vi "Acquire_PID_Tests_steps_gs.vi"() -> ()   [LabVIEW 2016]
uses:
  Globals/PressuresGlobal.vi
panel:
  in  "PID Time":dbl=20.0
  out "Current Set point":dbl
  out "Exp Time":dbl
  in  "Time_Stable(s)":dbl=20.0
  in  "Set Points":dbl[](array[numeric])=[0.1, 0.2, 0.3, 0.4, 0.5, 0.6, 0.7, 0.8, 0.9]
  in  "Wait For Microscope?":bool=TRUE
  in  "stop2":bool
  in  "Flow Path":path=path "E:/maggot images/Jacob/20171121/stepTest20units_run101.mat"
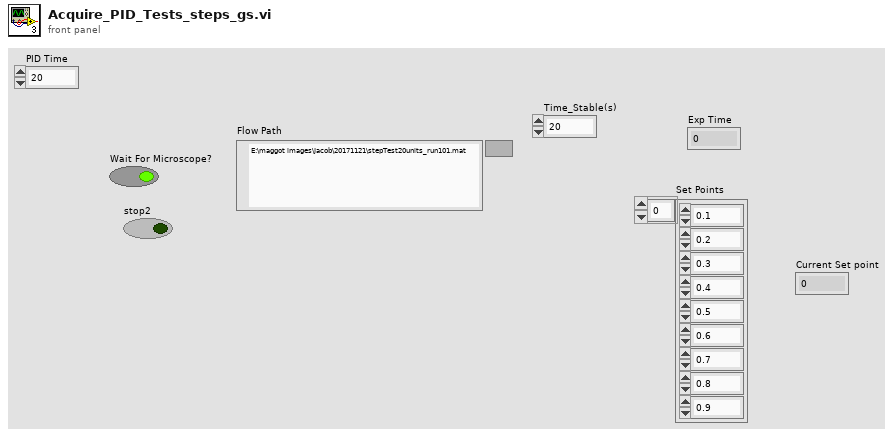
[diagram p1: front panel]
types:
  T1 = cluster{"relative seconds":dbl, "Pressures":dbl[], "F1 PID gains":dbl[], "FTot PID gains":dbl[], "PID On?":i16, "flow setpoints":dbl[]}
  T2 = cluster{"Time":dbl, "All Flow-Rates":dbl[], "Flow 2 Filter Time":dbl, "Flow 1 Filter Time":dbl}
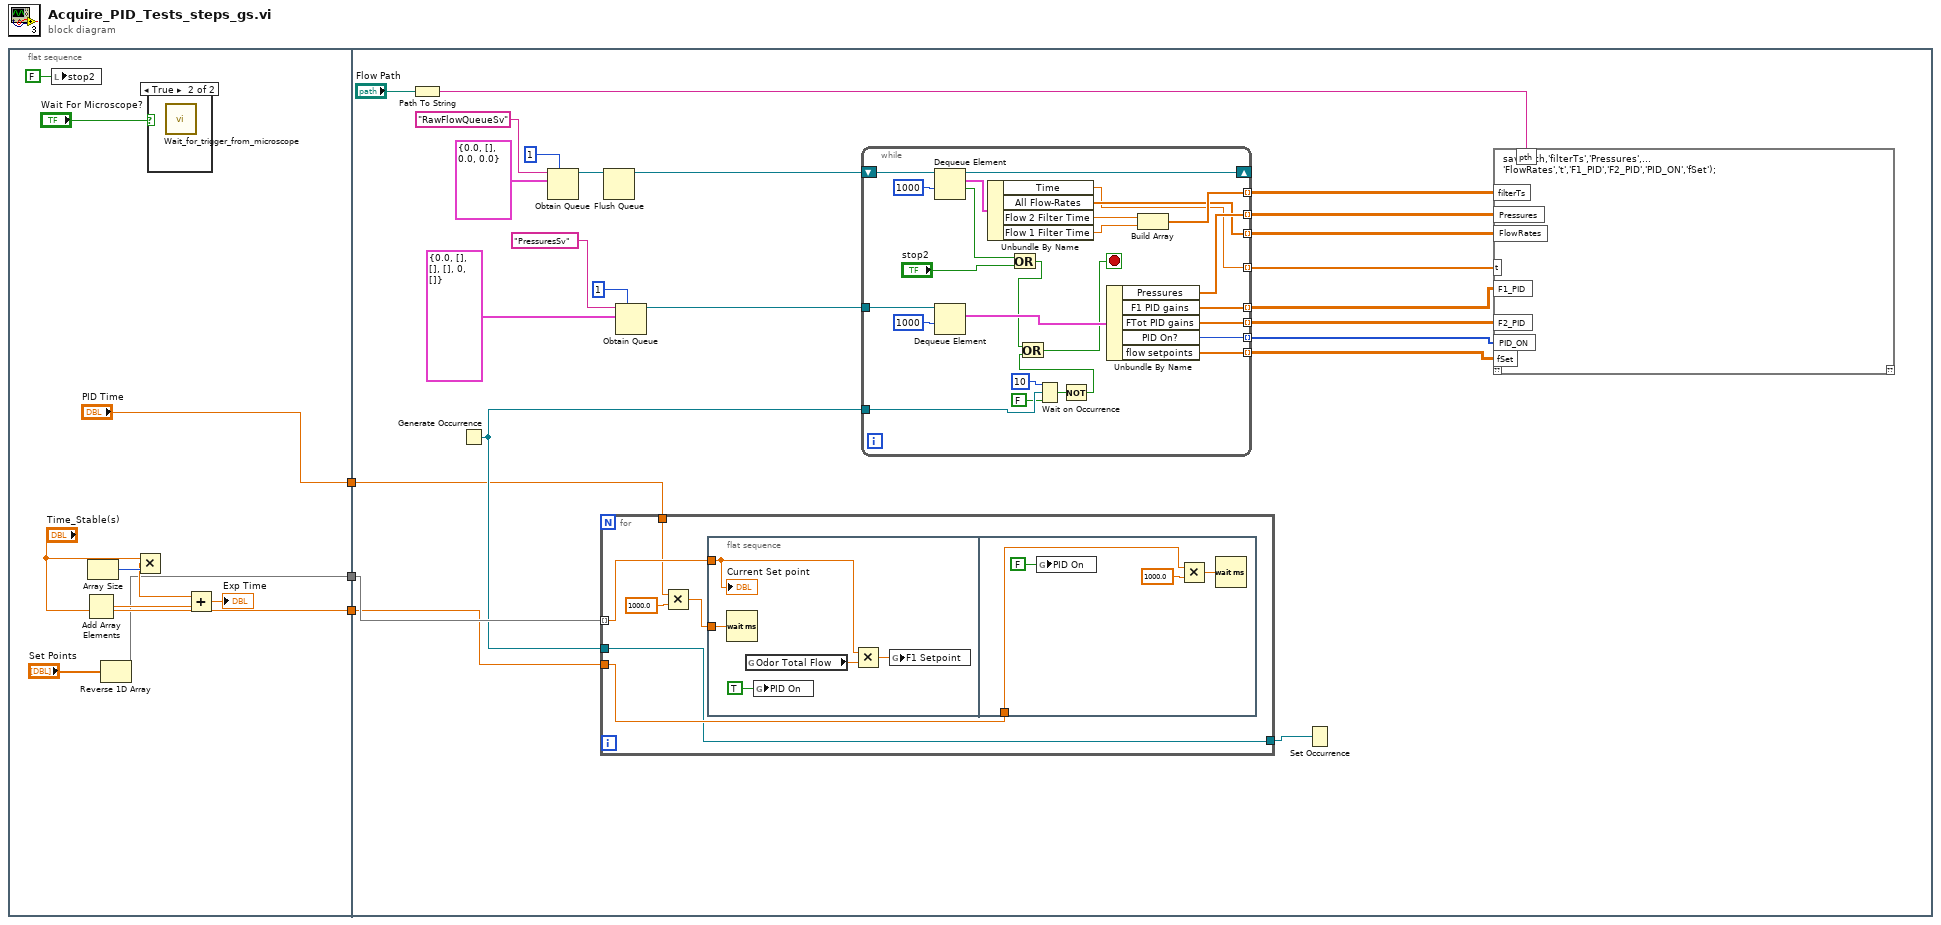
[diagram p0: block diagram]
diagram:
  n1 = flat-sequence {
    tunnel: [w5] -> w3
    tunnel: ["Time_Stable(s)"] -> w2
    tunnel: ["PID Time"] -> w1
    tunnel: w3 -> [w18]
    tunnel: w2 -> [w17]
    tunnel: w1 -> [w14]
    frame #0 {
      n2 = local write "stop2"(FALSE ("stop2")) -> ()
      n3 = Add Array Elements() -> (sum=w7:dbl)  [unwired: 1 in]
      n4 = Array Size() -> (size(s)=w9:i32)  [unwired: 1 in]
      n5 = Reverse 1D Array(array="Set Points") -> (reversed array=w5:dbl[])
      n6 = Multiply(x="Time_Stable(s)", y=w9) -> (x*y=w8:dbl)
      n7 = case shown="True" "Wait For Microscope?" {
        frame False {
        }
        frame True {
          n8 = call "Wait_for_trigger_from_microscope.vi"() -> ()  [unwired: 12 in]
        }
      }
      n9 = Add(x=w8, y=w7) -> (x+y=→"Exp Time":dbl)
    }
    frame #1 {
      n10 = Path To String(path="Flow Path") -> (string=w21:string)
      n11 = Generate Occurrence() -> (w16:refnum<k4>)
      n12 = Obtain Queue(max queue size (-1, unlimited)=1, name (unnamed)="RawFlowQueueSv", element data type=T2 {"Time"=0.0, "All Flow-Rates"=[], "Flow 2 Filter Time"=0.0, "Flow 1 Filter Time"=0.0} ("output cluster")) -> (queue out=w36:refnum<queue>)  [unwired: 2 in, 2 out]
      n13 = for {
        tunnel: w18 -> [w43] mode=indexing
        tunnel: w17 -> [w40]
        tunnel: w16 -> [w39]
        tunnel: [w39] -> w15
        tunnel: w14 -> [w38]
        n14 = Multiply(x=w38, y=1000.0) -> (x*y=w41:dbl)
        n15 = flat-sequence {
          tunnel: w43 -> [w47]
          tunnel: w41 -> [w45]
          tunnel: w40 -> [w50]
          frame #0 {
            n16 = Wait (ms)(milliseconds to wait=w45) -> ()  [unwired: 1 out]
            n17 = global read "PressuresGlobal.vi" "Odor Total Flow"() -> (w48:dbl)
            n18 = global write "PressuresGlobal.vi" "PID On"(TRUE ("PID On")) -> ()
            n19 = Multiply(x=w47, y=w48) -> (x*y=w46:dbl)
            n20 = global write "PressuresGlobal.vi" "F1 Setpoint"(w46) -> ()
            "Current Set point" <- w47
          }
          frame #1 {
            n21 = global write "PressuresGlobal.vi" "PID On"(FALSE ("PID On")) -> ()
            n22 = Multiply(x=w50, y=1000.0) -> (x*y=w51:dbl)
            n23 = Wait (ms)(milliseconds to wait=w51) -> ()  [unwired: 1 out]
          }
        }
      }
      n24 = Flush Queue(queue=w36) -> (queue out=w35:refnum<queue>)  [unwired: 1 in, 2 out]
      n25 = Obtain Queue(max queue size (-1, unlimited)=1, name (unnamed)="PressuresSv", element data type=T1 {"relative seconds"=0.0, "Pressures"=[], "F1 PID gains"=[], "FTot PID gains"=[], "PID On?"=0, "flow setpoints"=[]} ("output cluster")) -> (queue out=w31:refnum<queue>)  [unwired: 2 in, 2 out]
      n26 = while {
        shift-right: [w75] -> _
        shift-left: w35 -> [w78]
        tunnel: w31 -> [w72]
        tunnel: [w67] -> w22 mode=indexing
        tunnel: [w66] -> w23 mode=indexing
        tunnel: [w65] -> w24 mode=indexing
        tunnel: [w64] -> w26 mode=indexing
        tunnel: [w63] -> w28 mode=indexing
        tunnel: [w62] -> w27 mode=indexing
        tunnel: [w61] -> w25 mode=indexing
        tunnel: [w60] -> w19 mode=indexing
        tunnel: w16 -> [w59]
        stop <- w54 stop-if-true
        n27 = Dequeue Element(queue=w78, timeout in ms (-1)=1000) -> (queue out=w75:refnum<queue>, element=w71:T2, timed out?=w76:bool)  [unwired: 1 in, 1 out]
        n28 = Dequeue Element(queue=w72, timeout in ms (-1)=1000) -> (element=w68:T1)  [unwired: 1 in, 3 out]
        n29 = Unbundle By Name(w71) -> ("Time"=w61:dbl, "All Flow-Rates"=w62:dbl[], "Flow 2 Filter Time"=w70:dbl, "Flow 1 Filter Time"=w69:dbl)
        n30 = Or(x=w76, y="stop2") -> (x .or. y?=w55:bool)
        n31 = Wait on Occurrence(1:FALSE ("ignore previous (T)"), 2:w59, 3:10 ("ms timeout (-1)")) -> (0:w56:bool)
        n32 = Not(x=w56) -> (.not. x?=w53:bool)
        n33 = Or(x=w55, y=w53) -> (x .or. y?=w54:bool)
        n34 = Unbundle By Name(w68) -> ("Pressures"=w64:dbl[], "F1 PID gains"=w65:dbl[], "FTot PID gains"=w66:dbl[], "PID On?"=w67:i16, "flow setpoints"=w60:dbl[])
        n35 = Build Array(w70, w69) -> (w63:dbl[])
      }
      n36 = Set Occurrence(w15) -> ()
      n37 = script code="save(pth,'filterTs','Pressures',...\n'FlowRates','t','F1_PID','F2_PID','PID_ON','fSet');"("pth"=w21, "t"=w25, "F1_PID"=w24, "F2_PID"=w23, "PID_ON"=w22, "Pressures"=w26, "FlowRates"=w27, "filterTs"=w28, "fSet"=w19) -> ()  [unwired: 1 in, 1 out]
    }
  }
